vi "UE9 Low Latency Stream.vi"() -> ()   [LabVIEW 2021]
panel:
  in  "Delay [ms]":u32
  in  "FirstFound":bool=TRUE
  in  "ConnectionType":u16(ring) items=["LJ_ctUSB", "LJ_ctETHERNET"]
  in  "DeviceType":u16(ring)=1 items=["LJ_dtU3", "LJ_dtUE9"]
  in  "Address":string="192.168.1.209"
  out "Comm Backlog [%]":dbl format="%.2f"
  in  "Scans To Read Per Iteration":dbl=1.0 format="%.3f"
  out "UD Backlog [%]":dbl format="%.2f"
  out "Actual Scan Rate (Hz)":dbl=100.0 format="%.3f"
  out "# Scans Read":i32
  out "# of iterations":i32
  out "Data":dbl[][](array[numeric]) format="%.3f"
  in  "Scan Rate (Hz)":dbl=100.0 format="%.3f"
  in  "stop":bool
  out "Error Message":string
  # "Usually command/response is used in low-latency applications.  Stream is good at collecting data fast at precise intervals,\nbut is most efficient when it moves large chunks of data at a time.  This VI demonstrates techniques for moving small\nchunks of data more often."
  # "Specify an IP address for Ethernet, or Local ID\nfor USB.  If FirstFound is selected, Local ID is\nignored for USB.  Clear FirstFound if using Ethernet."
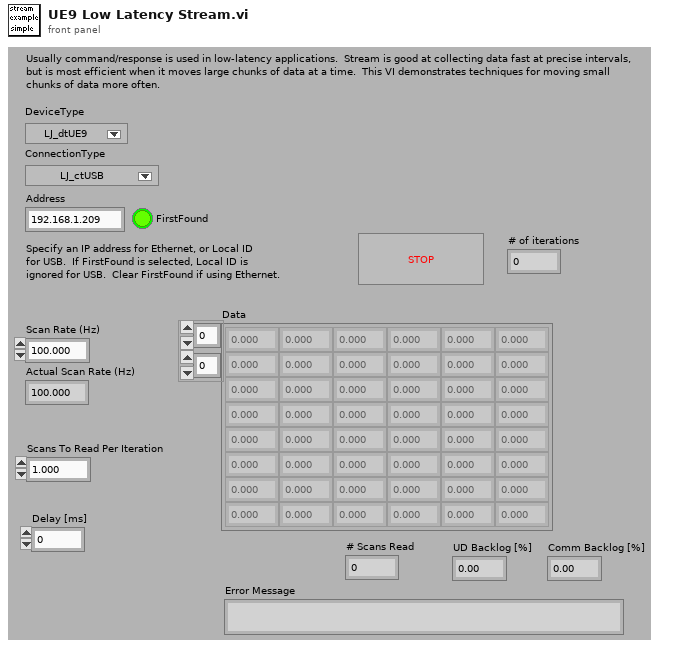
[diagram p1: front panel]
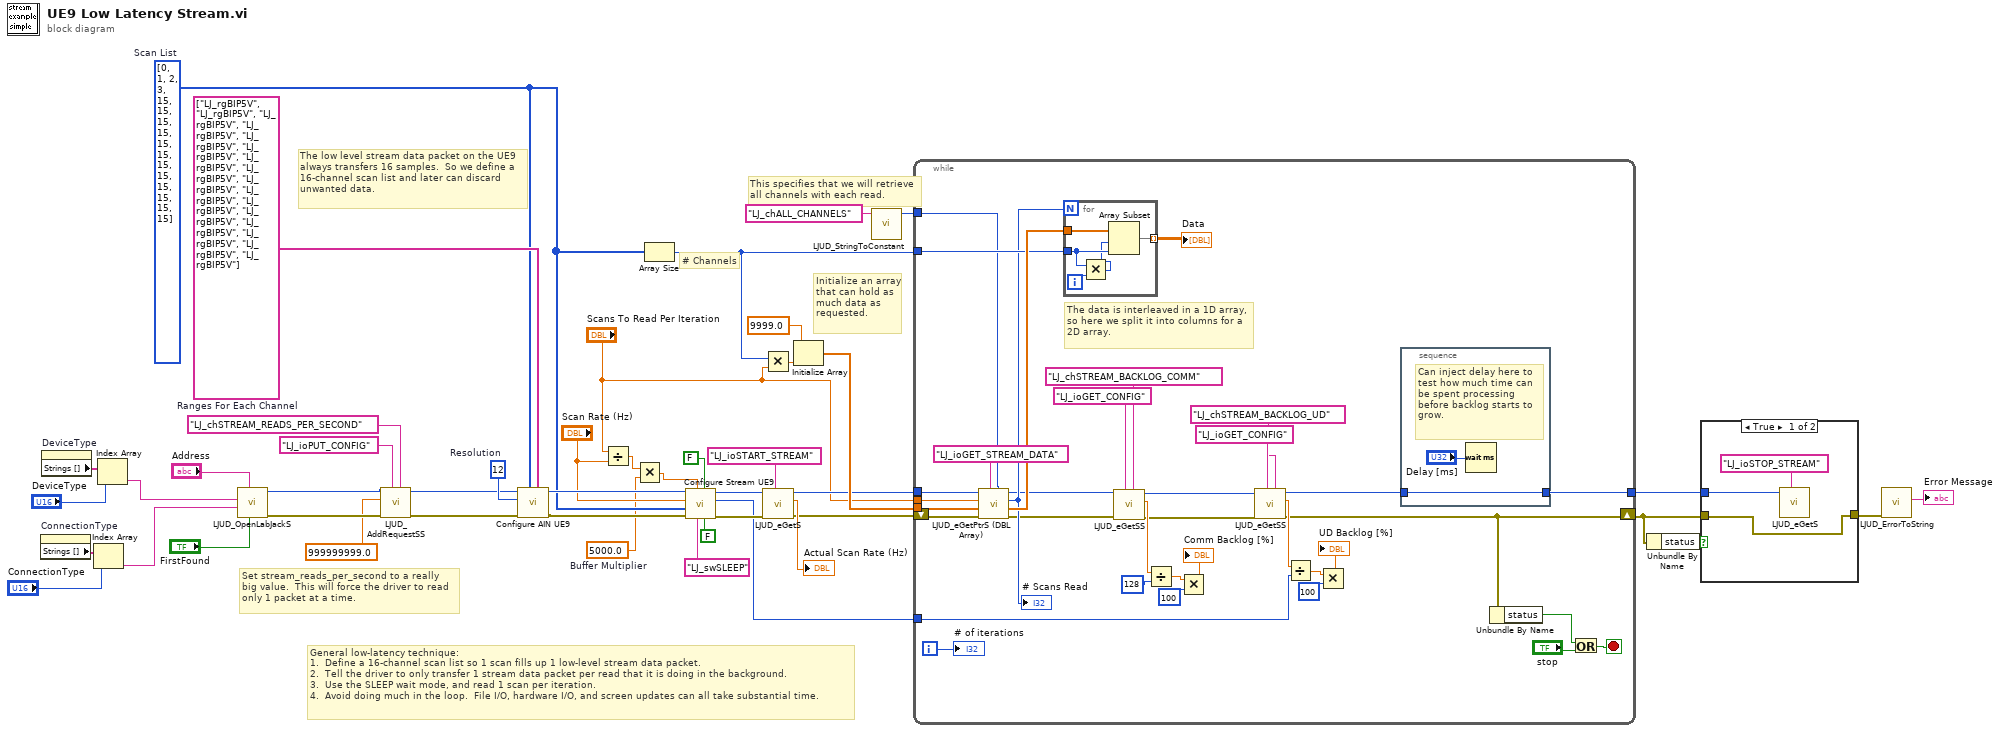
[diagram p0: block diagram]
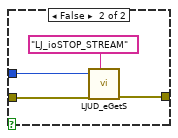
[diagram p2: hidden frame]
diagram:
  w9 = 5000.0  # Buffer Multiplier
  w24 = 12  # Resolution
  w25 = i32[] [0, 1, 2, 3, 15, 15, 15, 15, 15, 15, 15, 15, 15, 15, 15, 15]  # Scan List
  w26 = string[] ["LJ_rgBIP5V", "LJ_rgBIP5V", "LJ_rgBIP5V", "LJ_rgBIP5V", "LJ_rgBIP5V", "LJ_rgBIP5V", "LJ_rgBIP5V", "LJ_rgBIP5V", "LJ_rgBIP5V", "LJ_rgBIP5V", "LJ_rgBIP5V", "LJ_rgBIP5V", "LJ_rgBIP5V", "LJ_rgBIP5V", "LJ_rgBIP5V", "LJ_rgBIP5V"]  # Ranges For Each Channel
  # "General low-latency technique:\n1.  Define a 16-channel scan list so 1 scan fills up 1 low-level stream data packet.\n2.  Tell the driver to only transfer 1 stream data packet per read that it is doing in the background.\n3.  Use the SLEEP wait mode, and read 1 scan per iteration.\n4.  Avoid doing much in the loop.  File I/O, hardware I/O, and screen updates can all take substantial time."
  # "Set stream_reads_per_second to a really\nbig value.  This will force the driver to read\nonly 1 packet at a time."
  # "The low level stream data packet on the UE9\nalways transfers 16 samples.  So we define a\n16-channel scan list and later can discard\nunwanted data."
  # "Initialize an array\nthat can hold as\nmuch data as\nrequested."
  # "# Channels"
  # "This specifies that we will retrieve\nall channels with each read."
  n1 = property on="ConnectionType" class="Ring (strict)"() -> ("Strings []"=w7:string[])  [unwired: 2 in, 2 out]
  n2 = property on="DeviceType" class="Ring (strict)"() -> ("Strings []"=w8:string[])  [unwired: 2 in, 2 out]
  n3 = Index Array(array=w7, index="ConnectionType") -> (element=w2:string)
  n4 = Index Array(array=w8, index="DeviceType") -> (element=w1:string)
  n5 = call "LJUD_OpenLabJackS.vi"("FirstFound"="FirstFound", "Address"="Address", "ConnectionType"=w2, "DeviceType"=w1) -> ("error out"=w19:errorcluster, "Handle"=w18:i32)  [unwired: 5 in, 1 out]
  n6 = call "LJUD_AddRequestSS.vi"("Channel"="LJ_chSTREAM_READS_PER_SECOND" ("IOType"), "IOType"="LJ_ioPUT_CONFIG", "error in"=w19, "Value"=999999999.0, "Handle In"=w18) -> ("error out"=w17:errorcluster, "Handle Out"=w16:i32)  [unwired: 5 in]
  n7 = call "Configure AIN UE9.vi"("Ranges"=w26, "Channels"=w25, "error in"=w17, "Resolution"=w24, "Handle In"=w16) -> ("error out"=w32:errorcluster, "Handle Out"=w31:i32)  [unwired: 5 in]
  n8 = Divide(x="Scans To Read Per Iteration", y="Scan Rate (Hz)") -> (x/y=w13:dbl)
  n9 = Multiply(x=w13, y=w9) -> (x*y=w12:dbl)
  n10 = Array Size(array=w25) -> (size(s)=w40:i32)
  n11 = call "Configure Stream UE9.vi"("External Scan Trigger"=FALSE, "Scan Clock Output"=FALSE, "Wait Mode"="LJ_swSLEEP" ("Wait Mode (2)"), "PC buffer size (seconds)"=w12, "error in"=w32, "Scan List"=w25, "Scan Rate (Hz)"="Scan Rate (Hz)", "Handle In"=w31) -> ("error out"=w44:errorcluster, "PC buffer size (samples)"=w14:i32, "Handle Out"=w45:i32)  [unwired: 1 in]
  n12 = Multiply(x=w40, y="Scans To Read Per Iteration") -> (x*y=w43:dbl)
  n13 = call "LJUD_eGetS.vi"("IOType"="LJ_ioSTART_STREAM", "error in"=w44, "Handle In"=w45) -> ("error out"=w22:errorcluster, "Value Read"=→"Actual Scan Rate (Hz)":dbl, "Handle Out"=w30:i32)  [unwired: 6 in]
  n14 = Initialize Array(9999.0, w43) -> (w41:dbl[])
  n15 = call "LJUD_StringToConstant.vi"("String"="LJ_chALL_CHANNELS") -> ("Constant Number"=w27:i32)  [unwired: 9 in, 1 out]
  n16 = while {
    tunnel: w14 -> [w60]
    shift-left: w22 -> [w68]
    shift-right: [w61] -> w23
    tunnel: w27 -> [w71]
    tunnel: [w58] -> w38
    tunnel: w40 -> [w74]
    tunnel: w41 -> [w77]
    tunnel: "Scans To Read Per Iteration" -> [w75]
    tunnel: w30 -> [w79]
    i -> [w73]
    stop <- w70 stop-if-true
    # "The data is interleaved in a 1D array,\nso here we split it into columns for a\n2D array."
    n17 = call "LJUD_eGetPtrS (DBL Array).vi"("Channel"=w71, "IOType"="LJ_ioGET_STREAM_DATA", "error in"=w68, "DBL Array Write"=w77, "Value"=w75, "Handle In"=w79) -> ("error out"=w49:errorcluster, "DBL Array Read"=w76:dbl[], "Value"=w69:i32, "Handle Out"=w48:i32)  [unwired: 2 in]
    "# Scans Read" <- w69
    n18 = for {
      N: w69 -> [_]
      tunnel: w76 -> [w88]
      tunnel: w74 -> [w87]
      tunnel: [w84] -> w72 mode=indexing
      i -> [w86]
      n19 = Multiply(x=w87, y=w86) -> (x*y=w85:i32)
      n20 = Array Subset(array=w88, index=w85, length=w87) -> (w84:dbl[])
    }
    "Data" <- w72
    n21 = call "LJUD_eGetSS.vi"("Channel"="LJ_chSTREAM_BACKLOG_COMM", "IOType"="LJ_ioGET_CONFIG", "error in"=w49, "Handle In"=w48) -> ("error out"=w50:errorcluster, "Value Read"=w57:dbl, "Handle Out"=w51:i32)  [unwired: 5 in]
    n22 = Divide(x=w57, y=128) -> (x/y=w54:dbl)
    n23 = Multiply(x=w54, y=100) -> (x*y=→"Comm Backlog [%]":dbl)
    n24 = call "LJUD_eGetSS.vi"("Channel"="LJ_chSTREAM_BACKLOG_UD", "IOType"="LJ_ioGET_CONFIG", "error in"=w50, "Handle In"=w51) -> ("error out"=w61:errorcluster, "Value Read"=w63:dbl, "Handle Out"=w59:i32)  [unwired: 5 in]
    n25 = Divide(x=w63, y=w60) -> (x/y=w64:dbl)
    n26 = Multiply(x=w64, y=100) -> (x*y=→"UD Backlog [%]":dbl)
    n27 = stacked-sequence {
      tunnel: w59 -> [w83]
      tunnel: [w83] -> w58
      frame #0 {
        # "Can inject delay here to\ntest how much time can\nbe spent processing\nbefore backlog starts to\ngrow."
        n28 = Wait (ms)(milliseconds to wait="Delay [ms]") -> ()  [unwired: 1 out]
      }
    }
    n29 = Unbundle By Name(w61) -> ("status"=w80:bool)
    n30 = Or(x=w80, y="stop") -> (x .or. y?=w70:bool)
    "# of iterations" <- w73
  }
  n31 = Unbundle By Name(w23) -> ("status"=w29:bool)
  n32 = case shown="True" w29 {
    tunnel: w38 -> [w90 w94]
    tunnel: [w89 w93] -> w37
    tunnel: w23 -> [w89 w92]
    frame True {
      n33 = call "LJUD_eGetS.vi"("IOType"="LJ_ioSTOP_STREAM", "Handle In"=w90) -> ()  [unwired: 7 in, 3 out]
    }
    frame False {
      n34 = call "LJUD_eGetS.vi"("IOType"="LJ_ioSTOP_STREAM", "error in"=w92, "Handle In"=w94) -> ("error out"=w93:errorcluster)  [unwired: 6 in, 2 out]
    }
  }
  n35 = call "LJUD_ErrorToString.vi"("error in"=w37) -> ("String"=→"Error Message":string)  [unwired: 10 in]
